vi "construct.vi"(8 "error in (no error)":errorcluster, 9 "configuration name":string, 10 "load config file?":bool=TRUE, 11 "TrajectoryRK110428Fiber in":refnum<class "TrajectoryRK110428Fiber_Spiral.lvclass">) -> (0 "error out":errorcluster, 3 "TrajectoryRK110428Fiber out":refnum<class "TrajectoryRK110428Fiber_Spiral.lvclass">)   [LabVIEW 2010, in "TrajectoryRK110428Fiber_Spiral.lvclass"]
uses:
  TrajectoryRK110428Fiber_Spiral.lvclass
  TrajectoryMG100122GenericFPGA/TrajectoryMG100122GenericFPGA/TrajectoryMG100122GenericFPGA.lvclass
  TrajectoryRK110428Fiber_Spiral.lvclass/TrajectoryRK110428Fiber_Spiral.ctl
  FPGAWrapper/GenericFPGAWrapper/GenericFPGAWrapper/GenericFPGAWrapper.lvclass
  common/classes/GenericComponent/GenericComponent/GenericComponent.lvclass
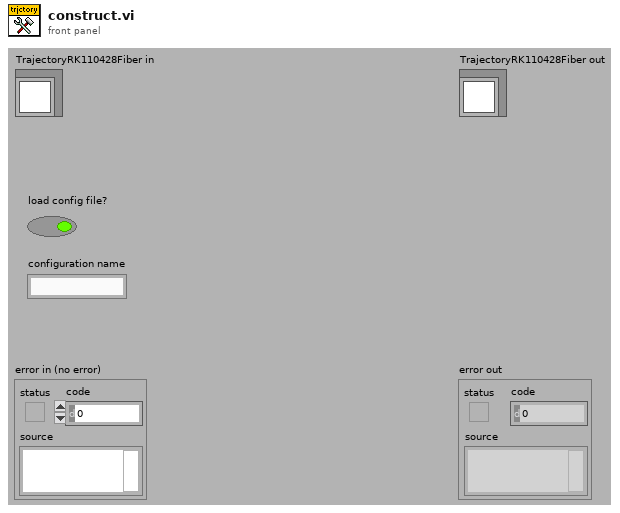
[diagram p1: front panel]
types:
  T1 = typedef "plugin_specification.ctl" = cluster{"class path":string, "configuration":string, "label":string, "settings name":string}
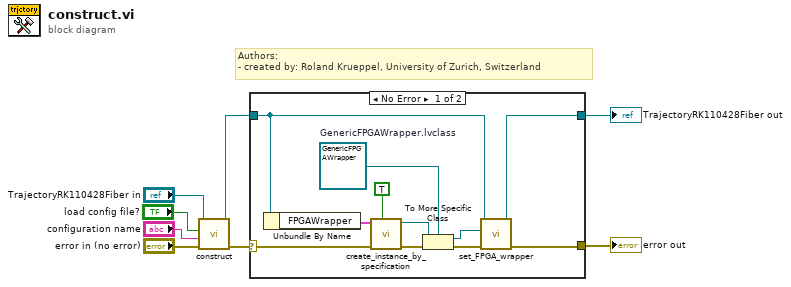
[diagram p0: block diagram]
diagram:
  # "Authors: \n- created by: Roland Krueppel, University of Zurich, Switzerland"
  n1 = call-parent "construct.vi"("error in (no error)"="error in (no error)", "configuration name"="configuration name", "load config file?"="load config file?", "GenericPlugin in"="TrajectoryRK110428Fiber in") -> ("error out"=w4:errorcluster, "GenericPlugin out"=w3:refnum<class "TrajectoryRK110428Fiber_Spiral.lvclass">)  [unwired: 6 in]
  n2 = case shown="No Error" w4 {
    selector: w4 -> [w18 w21]
    tunnel: w3 -> [w12 w20]
    tunnel: [w10 w20] -> w2
    tunnel: [w9 w21] -> w1
    frame No Error {
      w14 = refnum<class "GenericFPGAWrapper.lvclass"> refnum  # GenericFPGAWrapper.lvclass
      n3 = Unbundle By Name(w12) -> ("FPGAWrapper"=w19:T1)
      n4 = call "create_instance_by_specification.vi"("call constructor?"=TRUE, "error in (no error)"=w18, "component specification"=w19) -> ("error out"=w17:errorcluster, "GenericPlugin out"=w16:refnum<class "GenericComponent.lvclass">)  [unwired: 6 in, 1 out]
      n5 = To More Specific Class(target class=w14, reference=w16, error in=w17) -> (specific class reference=w11:refnum<class "GenericFPGAWrapper.lvclass">, error out=w13:errorcluster)
      n6 = call-dynamic "set_FPGA_wrapper.vi"("error in (no error)"=w13, "GenericFPGAWrapper.lvclass"=w11, "TrajectoryMG100122GenericFPGA in"=w12) -> ("error out"=w9:errorcluster, "TrajectoryMG100122GenericFPGA out"=w10:refnum<class "TrajectoryRK110428Fiber_Spiral.lvclass">)  [unwired: 7 in]
    }
    frame Error {
    }
  }
  "error out" <- w1
  "TrajectoryRK110428Fiber out" <- w2
